vi "Delete_Signal.vi"(10 "CAN_MSGs":T1={"Scaling Factor"=1, "Physical value"=0.0, "CAN_Frames"={"CAN_ID"=0, "MSGTYPE"=128, "Payload"=[], "Length"=0}, "Offset value"=0.0, "Framing datas"=[], "CAN_Frame Enable"=FALSE, "Add Signal"=FALSE, "Delete Signal"=FALSE, "Signal Values"=[], "Time(ms)"=0.0, "Repetition"=FALSE, "Delay"=FALSE, "Delay time"=0.0} {"CAN_Frames"."Payload" format="%.0x"; "CAN_Frames"."MSGTYPE" items=["STATUS"=128, "EXTENDED"=2, "RTR"=1, "DATA MSG"=0]; "CAN_Frames"."CAN_ID" format="%.0x"}) -> (2 "CAN_MSGs 2":T1={"Scaling Factor"=1, "Physical value"=0.0, "CAN_Frames"={"CAN_ID"=0, "MSGTYPE"=128, "Payload"=[], "Length"=0}, "Offset value"=0.0, "Framing datas"=[], "CAN_Frame Enable"=FALSE, "Add Signal"=FALSE, "Delete Signal"=FALSE, "Signal Values"=[], "Time(ms)"=0.0, "Repetition"=FALSE, "Delay"=FALSE, "Delay time"=0.0} {"CAN_Frames"."Payload" format="%.0x"; "CAN_Frames"."MSGTYPE" items=["STATUS"=128, "EXTENDED"=2, "RTR"=1, "DATA MSG"=0]; "CAN_Frames"."CAN_ID" format="%.0x"})   [LabVIEW 2024, in "PCANusb_DTU.lvlib"]
uses:
  PCANusb_DTU.lvlib
  CAN_MSGs.ctl
  CAN_Frames_ctrl.ctl
  Framing datas.ctl
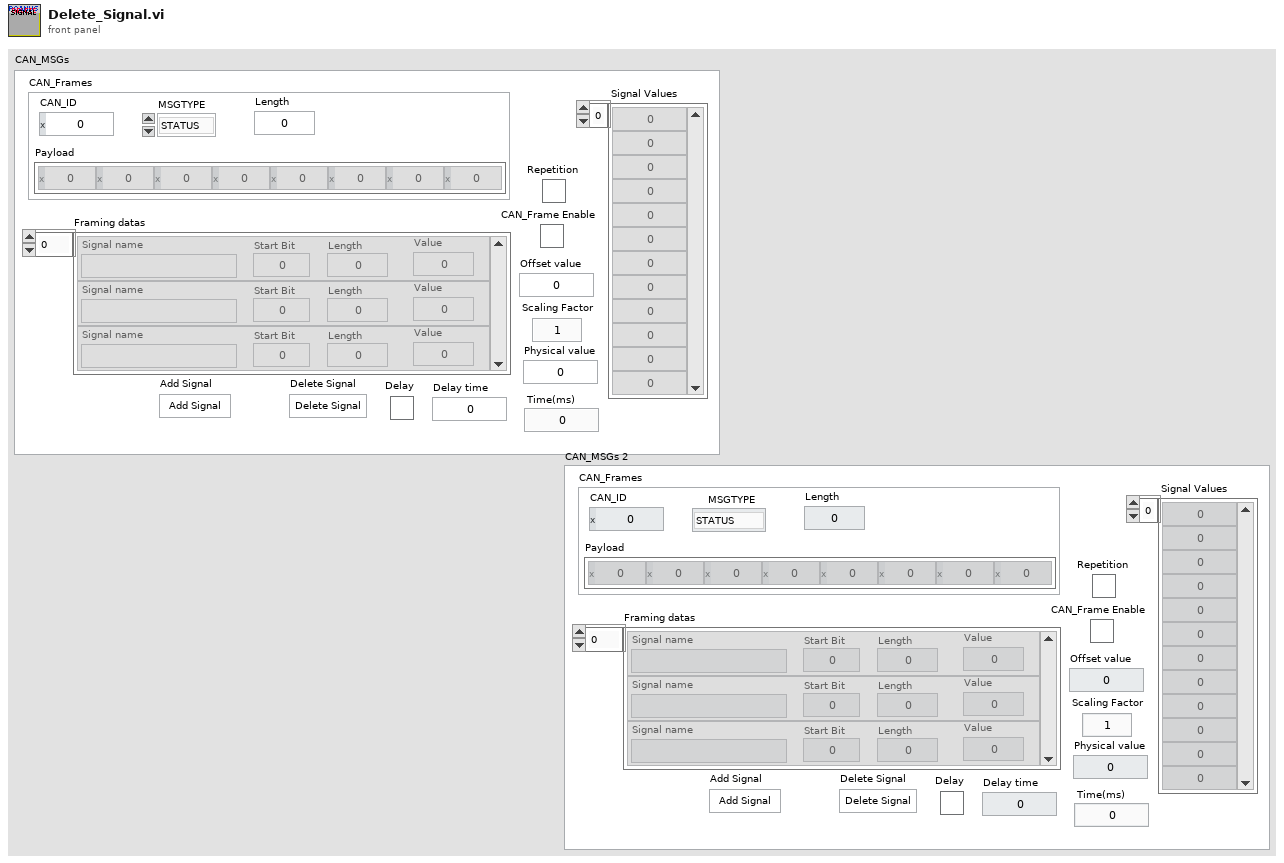
[diagram p1: front panel]
types:
  T1 = typedef "PCANusb_DTU.lvlib/CAN_MSGs.ctl" = cluster{"Scaling Factor":u16, "Physical value":dbl, "CAN_Frames":T2, "Offset value":dbl, "Framing datas":T3[], "CAN_Frame Enable":bool, "Add Signal":bool, "Delete Signal":bool, "Signal Values":dbl[], "Time(ms)":dbl, "Repetition":bool, "Delay":bool, "Delay time":dbl}
  T2 = typedef "PCANusb_DTU.lvlib/CAN_Frames_ctrl.ctl" = cluster{"CAN_ID":u32, "MSGTYPE":u8, "Payload":u8[], "Length":u8}
  T3 = typedef "PCANusb_DTU.lvlib/Framing datas.ctl" = cluster{"Signal name":string, "Start Bit":u8, "Length":u8, "Value":u16}
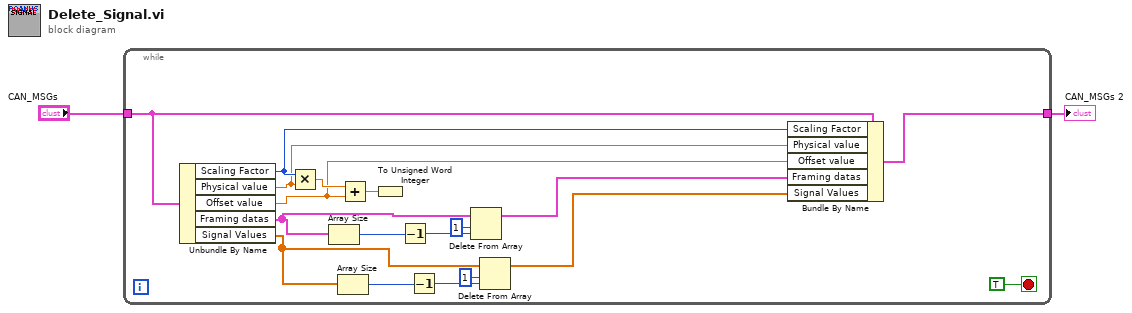
[diagram p0: block diagram]
diagram:
  n1 = while {
    tunnel: "CAN_MSGs" -> [w19]
    tunnel: [w16] -> w1
    stop <- TRUE stop-if-true
    n2 = Unbundle By Name(w19) -> ("Scaling Factor"=w15:u16, "Physical value"=w14:dbl, "Offset value"=w13:dbl, "Framing datas"=w11:T3[], "Signal Values"=w9:dbl[])
    n3 = Multiply(x=w15, y=w14) -> (x*y=w18:dbl)
    n4 = Array Size(array=w11) -> (size(s)=w12:i32)
    n5 = Array Size(array=w9) -> (size(s)=w10:i32)
    n6 = Add(x=w18, y=w13) -> (x+y=w17:dbl)
    n7 = To Unsigned Word Integer(number=w17) -> ()  [unwired: 1 out]
    n8 = Decrement(x=w12) -> (x-1=w6:i32)
    n9 = Decrement(x=w10) -> (x-1=w5:i32)
    n10 = Delete From Array(array=w11, length=1, index=w6) -> (array with subset deleted=w4:T3[])  [unwired: 1 out]
    n11 = Delete From Array(array=w9, length=1, index=w5) -> (array with subset deleted=w3:dbl[])  [unwired: 1 out]
    n12 = Bundle By Name(cluster=w19, "Scaling Factor"=w15, "Physical value"=w14, "Offset value"=w13, "Framing datas"=w4, "Signal Values"=w3) -> (w16:T1)
  }
  "CAN_MSGs 2" <- w1
